vi "ST_parse_reference_data.vi"(4 "reference_name":string, 6 "recordset_data":variant[][](array[variant]), 8 "error_in":errorcluster, 11 "command_nmb":u8) -> (0 "error_out":errorcluster, 3 "reference_data_to_PLC":u8[](array[numeric]))   [LabVIEW 2020]
uses:
  ST_reference_info.ctl
  _misc/byte_array_parser/from_I16.vi
  reference_byte_offsset/ref_INT_offset.vi
  _misc/byte_array_parser/from_SGL.vi
  reference_byte_offsset/ref_REAL_offset.vi
  _misc/byte_array_parser/from_STR_to_PLC_STRING[50].vi
  reference_byte_offsset/ref_STRING_offset.vi
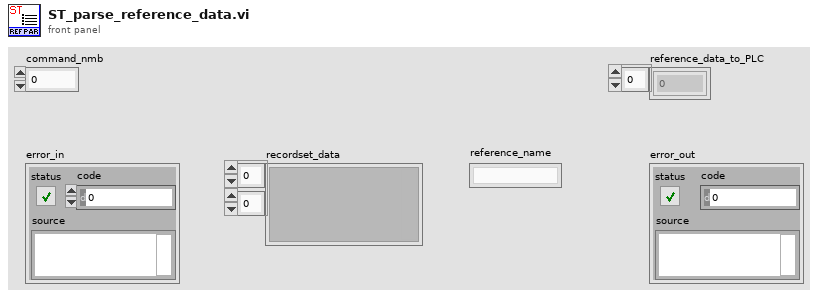
[diagram p1: front panel]
types:
  T1 = typedef "ST_reference_info.ctl" = cluster{"INT_number":i32, "REAL_number":i32, "STRING_number":i32, "STRING_size":i32, "BYTE_array":u8[]}
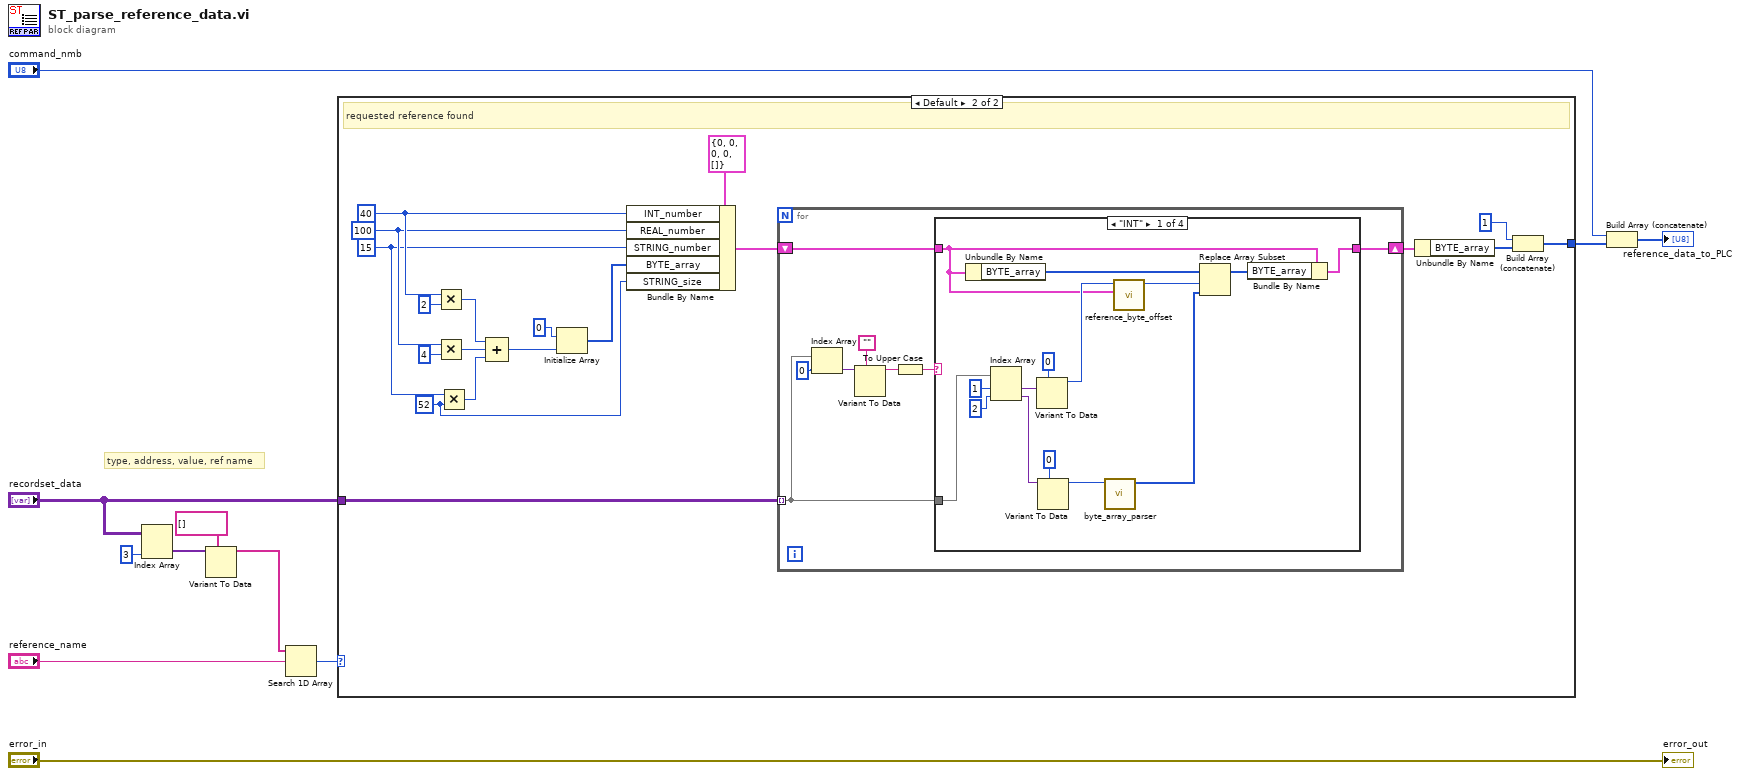
[diagram p0: block diagram]
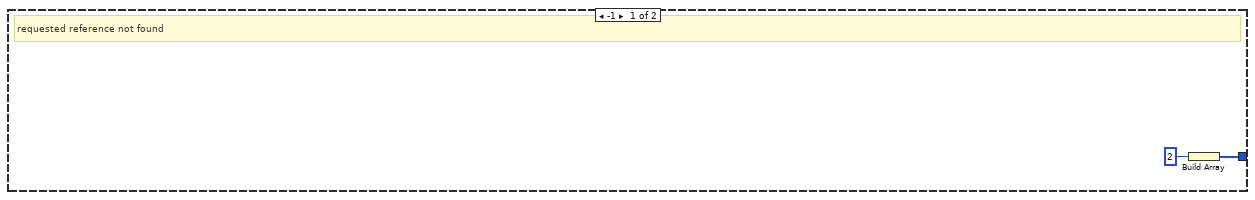
[diagram p2: hidden frame]
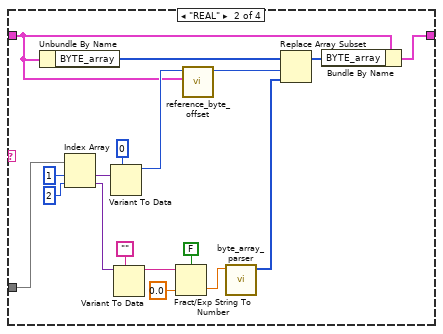
[diagram p3: hidden frame]
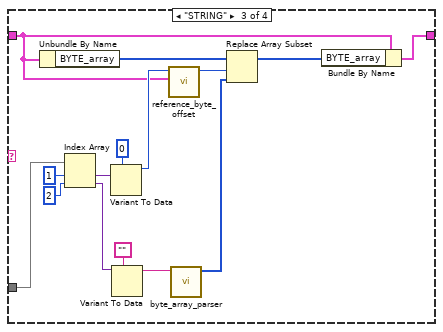
[diagram p4: hidden frame]
diagram:
  # "type, address, value, ref name"
  n1 = Index Array(array="recordset_data", index (col)=3 ("disabled index (col)")) -> (element=w5:variant[])  [unwired: 1 in]
  n2 = Variant To Data(type=string[] [], Variant=w5) -> (data=w4:string[])  [unwired: 1 in, 1 out]
  n3 = Search 1D Array(1D array=w4, element="reference_name") -> (index of element=w2:i32)  [unwired: 1 in]
  n4 = case shown="Default" w2 {
    tunnel: [w12 w16] -> w11
    tunnel: "recordset_data" -> [_ w17]
    frame -1 {
      # "requested reference not found"
      n5 = Build Array(u8 2) -> (w12:u8[])
    }
    frame Default {
      w18 = 52 ("y")
      w19 = 15 ("STRING_number")
      w20 = 100 ("REAL_number")
      w21 = 40 ("INT_number")
      # "requested reference found"
      n6 = Multiply(x=w21, y=2) -> (x*y=w26:i32)
      n7 = Multiply(x=w20, y=4) -> (x*y=w25:i32)
      n8 = Multiply(x=w19, y=w18) -> (x*y=w24:i32)
      n9 = Compound Arithmetic op=unknown(w26, w25, w24) -> (w23:i32)
      n10 = Initialize Array(u8 0 ("element"), w23) -> (w29:u8[])
      n11 = Bundle By Name(cluster=T1 {"INT_number"=0, "REAL_number"=0, "STRING_number"=0, "STRING_size"=0, "BYTE_array"=[]}, "INT_number"=w21, "REAL_number"=w20, "STRING_number"=w19, "BYTE_array"=w29, "STRING_size"=w18) -> (w31:T1)
      n12 = for {
        tunnel: w17 -> [w34] mode=indexing
        shift-right: [w33] -> w22
        shift-left: w31 -> [w40]
        n13 = Index Array(array=w34, index=0) -> (element=w38:variant)
        n14 = Variant To Data(type="", Variant=w38) -> (data=w36:string)  [unwired: 1 in, 1 out]
        n15 = To Upper Case(1:w36) -> (0:w35:string)
        n16 = case shown="\"INT\"" w35 {
          tunnel: w40 -> [w41 w62 w74 w89]
          tunnel: w34 -> [w55 w73 w88 _]
          tunnel: [w47 w66 w80 w89] -> w33
          frame "INT" {
            n17 = Unbundle By Name(w41) -> ("BYTE_array"=w49:u8[])
            n18 = Index Array(array=w55, index #1=1 ("index"), index #2=2 ("index")) -> (element #1=w52:variant, element #2=w50:variant)
            n19 = Variant To Data(type=i16 0 ("index"), Variant=w52) -> (data=w43:i16)  [unwired: 1 in, 1 out]
            n20 = Variant To Data(type=i16 0 ("index"), Variant=w50) -> (data=w45:i16)  [unwired: 1 in, 1 out]
            n21 = call-poly "byte_array_parser.vi"("I16"=w45) -> ("byte_array"=w44:u8[])  [unwired: 9 in, 1 out]
            n22 = call-poly "reference_byte_offset.vi"("ST_reference_info"=w41, "INT_position"=w43) -> ("reference_byte_array_offset"=w42:i32)  [unwired: 9 in]
            n23 = Replace Array Subset(array=w49, new element=w44, index=w42) -> (w48:u8[])
            n24 = Bundle By Name(cluster=w41, "BYTE_array"=w48) -> (w47:T1)
          }
          frame "REAL" {
            n25 = Unbundle By Name(w62) -> ("BYTE_array"=w68:u8[])
            n26 = Index Array(array=w73, index #1=1 ("index"), index #2=2 ("index")) -> (element #1=w70:variant, element #2=w61:variant)
            n27 = Variant To Data(type=i16 0 ("index"), Variant=w70) -> (data=w64:i16)  [unwired: 1 in, 1 out]
            n28 = Variant To Data(type="", Variant=w61) -> (data=w59:string)  [unwired: 1 in, 1 out]
            n29 = Fract/Exp String To Number(use system decimal point (T)=FALSE, string=w59, default (0 dbl)=sgl 0.0 ("index")) -> (number=w57:sgl)  [unwired: 1 in, 1 out]
            n30 = call-poly "reference_byte_offset.vi"("ST_reference_info"=w62, "REAL_position"=w64) -> ("reference_byte_array_offset"=w63:i32)  [unwired: 9 in]
            n31 = call-poly "byte_array_parser.vi"("I16"=w57) -> ("byte_array"=w65:u8[])  [unwired: 9 in, 1 out]
            n32 = Replace Array Subset(array=w68, new element=w65, index=w63) -> (w67:u8[])
            n33 = Bundle By Name(cluster=w62, "BYTE_array"=w67) -> (w66:T1)
          }
          frame "STRING" {
            n34 = Unbundle By Name(w74) -> ("BYTE_array"=w82:u8[])
            n35 = Index Array(array=w88, index #1=1 ("index"), index #2=2 ("index")) -> (element #1=w85:variant, element #2=w83:variant)
            n36 = Variant To Data(type=i16 0 ("index"), Variant=w85) -> (data=w76:i16)  [unwired: 1 in, 1 out]
            n37 = Variant To Data(type="", Variant=w83) -> (data=w78:string)  [unwired: 1 in, 1 out]
            n38 = call-poly "reference_byte_offset.vi"("ST_reference_info"=w74, "STRING_position"=w76) -> ("reference_byte_array_offset"=w75:i32)  [unwired: 9 in]
            n39 = call-poly "byte_array_parser.vi"("String"=w78) -> ("byte_array"=w77:u8[])  [unwired: 9 in, 1 out]
            n40 = Replace Array Subset(array=w82, new element=w77, index=w75) -> (w81:u8[])
            n41 = Bundle By Name(cluster=w74, "BYTE_array"=w81) -> (w80:T1)
          }
          frame Default {
          }
        }
      }
      n42 = Unbundle By Name(w22) -> ("BYTE_array"=w15:u8[])
      n43 = Build Array (concatenate)(u8 1, w15) -> (w16:u8[])
    }
  }
  n44 = Build Array (concatenate)("command_nmb", w11) -> (→"reference_data_to_PLC":u8[])
  "error_out" <- "error_in"
